vi "profibus to tag bus.vi"(9 "Data in":u8[](array[numeric]), 10 "slave configuration":T2, 11 "data table in":T1) -> (3 "data table out":T1)   [LabVIEW 2013, in "Profibus Module runtime.lvclass"]
uses:
  Profibus Module runtime.lvclass
  profibus slave configuration.ctl
  profibus mapping configuration.ctl
  <vilib>/NI/Tag Bus/tag/Data Type.ctl
  <vilib>/NI/Tag Bus/table/data table.ctl
  <vilib>/NI/Tag Bus/table/data polymorphs/write one/write Double.vi
  <vilib>/NI/Tag Bus/table/data polymorphs/write one/write Array of U8.vi
  <vilib>/NI/Tag Bus/table/data polymorphs/write one/write Single.vi
  <vilib>/NI/Tag Bus/table/data polymorphs/write one/write I32.vi
  <vilib>/NI/Tag Bus/table/data polymorphs/write one/write U32.vi
  <vilib>/NI/Tag Bus/table/data polymorphs/write one/write U16.vi
  <vilib>/NI/Tag Bus/table/data polymorphs/write one/write I16.vi
  <vilib>/NI/Tag Bus/table/data polymorphs/write one/write U8.vi
  <vilib>/NI/Tag Bus/table/data polymorphs/write one/write I8.vi
  <vilib>/NI/Tag Bus/table/data polymorphs/write one/write Boolean.vi
  <vilib>/NI/Tag Bus/table/data table.lvlib
  <vilib>/NI/Tag Bus/tag/tag descriptor.lvclass
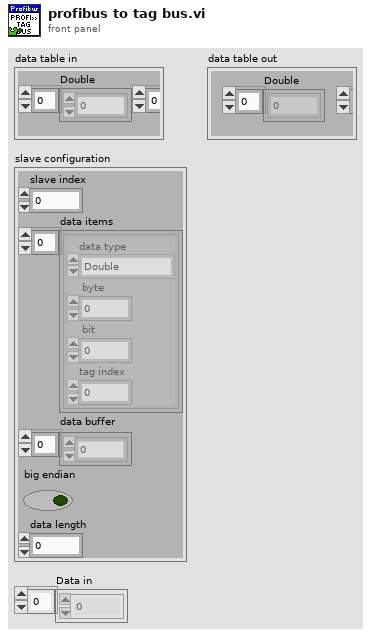
[diagram p1: front panel]
types:
  T1 = typedef "tag bus.lvlib/data table.lvlib/data table.ctl" = cluster{"Double":dbl[], "Single":sgl[], "I64":i64[], "I32":i32[], "I16":i16[], "I8":i8[], "U64":u64[], "U32":u32[], "U16":u16[], "U8":u8[], "Boolean":bool[], "String":string[], "Array of Double":cluster{"DBL Array":dbl[]}[], "Array of Single":cluster{"SGL Array":sgl[]}[], "Array of I64":cluster{"I64 Array":i64[]}[], "Array of I32":cluster{"I32 Array":i32[]}[], "Array of I16":cluster{"I16 Array":i16[]}[], "Array of I8":cluster{"I8 Array":i8[]}[], "Array of U64":cluster{"U64 Array":u64[]}[], "Array of U32":cluster{"U32 Array":u32[]}[], "Array of U16":cluster{"U16 Array":u16[]}[], "Array of U8":cluster{"U8 Array":u8[]}[], "Array of Boolean":cluster{"Boolean Array":bool[]}[], "Array of String":cluster{"String Array":string[]}[]}
  T2 = typedef "Profibus Module runtime.lvclass/profibus slave configuration.ctl" = cluster{"slave index":i8, "data items":T3[], "data buffer":u8[], "big endian":bool, "data length":i32}
  T3 = typedef "Profibus Module runtime.lvclass/profibus mapping configuration.ctl" = cluster{"data type":T4, " byte":i32, " bit":i32, "tag index":i32}
  T4 = typedef "tag bus.lvlib/tag descriptor.lvclass/Data Type.ctl" = enum16{"Double", "Single", "I64", "I32", "I16", "I8", "U64", "U32", "U16", "U8", "Boolean", "String", "Array of Double", "Array of Single", "Array of I64", "Array of I32", "Array of I16", "Array of I8", "Array of U64", "Array of U32", "Array of U16", "Array of U8", "Array of Boolean", "Array of String"}
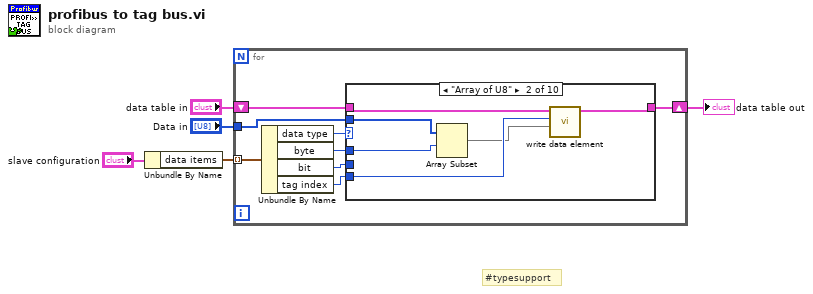
[diagram p0: block diagram]
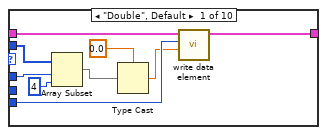
[diagram p2: hidden frame]
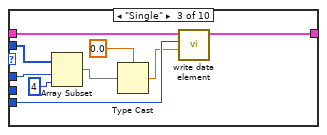
[diagram p3: hidden frame]
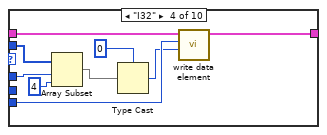
[diagram p4: hidden frame]
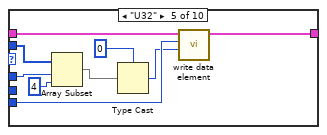
[diagram p5: hidden frame]
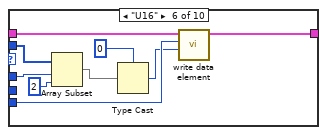
[diagram p6: hidden frame]
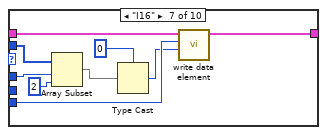
[diagram p7: hidden frame]
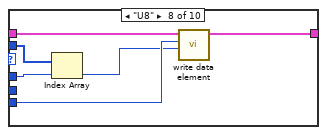
[diagram p8: hidden frame]
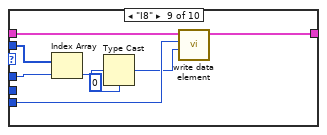
[diagram p9: hidden frame]
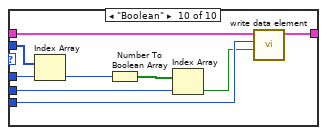
[diagram p10: hidden frame]
diagram:
  # "#typesupport"
  n1 = Unbundle By Name("slave configuration") -> ("data items"=w4:T3[])
  n2 = for {
    tunnel: w4 -> [w13] mode=indexing
    tunnel: "Data in" -> [w10]
    shift-right: [w7] -> w2
    shift-left: "data table in" -> [w6]
    n3 = Unbundle By Name(w13) -> ("data type"=w12:T4, "byte"=w11:i32, "bit"=w9:i32, "tag index"=w8:i32)
    n4 = case shown="\"Array of U8\"" w12 {
      tunnel: w10 -> [w22 w26 w37 w46 w55 w64 w73 w79 w87 w96]
      tunnel: w11 -> [w21 w25 w36 w45 w54 w63 w72 w78 w86 w95]
      tunnel: w9 -> [_ _ _ _ _ _ _ _ _ w92]
      tunnel: w8 -> [w17 w24 w32 w41 w50 w59 w68 w77 w85 w89]
      tunnel: [w15 w27 w30 w39 w48 w57 w66 w76 w84 w91] -> w7
      tunnel: w6 -> [w14 w28 w29 w38 w47 w56 w65 w75 w83 w90]
      frame "Double", Default {
        n5 = Array Subset(array=w22, index=w21, length=4) -> (w19:u8[])
        n6 = Type Cast(type=sgl 0.0, x=w19) -> (*(type *) &x=w16:sgl)
        n7 = call-poly <vilib>:"write data element.vi"("value"=w16, "index"=w17, "data table in"=w14) -> ("data table out"=w15:T1)  [unwired: 8 in]
      }
      frame "Array of U8" {
        n8 = Array Subset(array=w26, index=w25) -> (w23:u8[])  [unwired: 1 in]
        n9 = call-poly <vilib>:"write data element.vi"("value"=w23, "index"=w24, "data table in"=w28) -> ("data table out"=w27:T1)  [unwired: 8 in]
      }
      frame "Single" {
        n10 = Array Subset(array=w37, index=w36, length=4) -> (w34:u8[])
        n11 = Type Cast(type=sgl 0.0, x=w34) -> (*(type *) &x=w31:sgl)
        n12 = call-poly <vilib>:"write data element.vi"("value"=w31, "index"=w32, "data table in"=w29) -> ("data table out"=w30:T1)  [unwired: 8 in]
      }
      frame "I32" {
        n13 = Array Subset(array=w46, index=w45, length=4) -> (w43:u8[])
        n14 = Type Cast(type=0, x=w43) -> (*(type *) &x=w40:i32)
        n15 = call-poly <vilib>:"write data element.vi"("value"=w40, "index"=w41, "data table in"=w38) -> ("data table out"=w39:T1)  [unwired: 8 in]
      }
      frame "U32" {
        n16 = Array Subset(array=w55, index=w54, length=4) -> (w52:u8[])
        n17 = Type Cast(type=u32 0, x=w52) -> (*(type *) &x=w49:u32)
        n18 = call-poly <vilib>:"write data element.vi"("value"=w49, "index"=w50, "data table in"=w47) -> ("data table out"=w48:T1)  [unwired: 8 in]
      }
      frame "U16" {
        n19 = Array Subset(array=w64, index=w63, length=2) -> (w61:u8[])
        n20 = Type Cast(type=u16 0, x=w61) -> (*(type *) &x=w58:u16)
        n21 = call-poly <vilib>:"write data element.vi"("value"=w58, "index"=w59, "data table in"=w56) -> ("data table out"=w57:T1)  [unwired: 8 in]
      }
      frame "I16" {
        n22 = Array Subset(array=w73, index=w72, length=2) -> (w70:u8[])
        n23 = Type Cast(type=i16 0, x=w70) -> (*(type *) &x=w67:i16)
        n24 = call-poly <vilib>:"write data element.vi"("value"=w67, "index"=w68, "data table in"=w65) -> ("data table out"=w66:T1)  [unwired: 8 in]
      }
      frame "U8" {
        n25 = Index Array(array=w79, index=w78) -> (element=w74:u8)
        n26 = call-poly <vilib>:"write data element.vi"("value"=w74, "index"=w77, "data table in"=w75) -> ("data table out"=w76:T1)  [unwired: 8 in]
      }
      frame "I8" {
        n27 = Index Array(array=w87, index=w86) -> (element=w82:u8)
        n28 = Type Cast(type=i8 0, x=w82) -> (*(type *) &x=w81:i8)
        n29 = call-poly <vilib>:"write data element.vi"("value"=w81, "index"=w85, "data table in"=w83) -> ("data table out"=w84:T1)  [unwired: 8 in]
      }
      frame "Boolean" {
        n30 = Index Array(array=w96, index=w95) -> (element=w94:u8)
        n31 = Number To Boolean Array(number=w94) -> (Boolean array=w93:bool[])
        n32 = Index Array(array=w93, index=w92) -> (element=w88:bool)
        n33 = call-poly <vilib>:"write data element.vi"("value"=w88, "index"=w89, "data table in"=w90) -> ("data table out"=w91:T1)  [unwired: 8 in]
      }
    }
  }
  "data table out" <- w2
